vi "Launch Search.vi"(11 "Search Context":T1) -> (0 "error out":errorcluster)   [LabVIEW 2020, in "Better Search.lvlib" / "BetterSearch.lvclass"]
uses:
  BetterSearch.lvclass
  Data Types/Search Context.ctl
  Data Types/Start Search Type.ctl
  Data Types/Type Reflection Item.ctl
  Data Types/Context Comms.ctl
  Better Search.lvlib
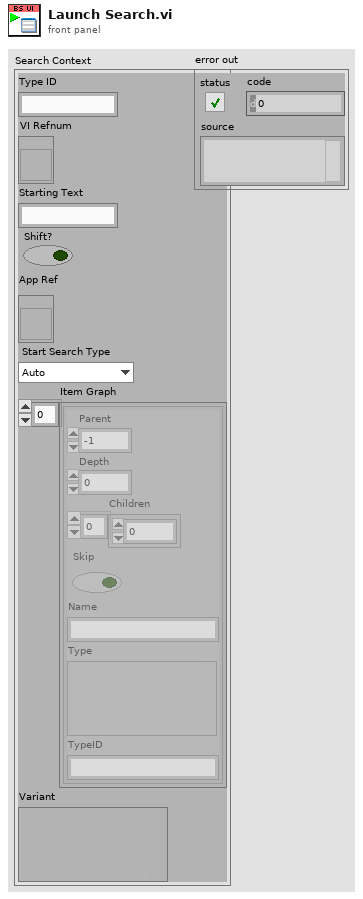
[diagram p1: front panel]
types:
  T1 = typedef "Better Search.lvlib/Search Context.ctl" = cluster{"Type ID":string, "VI Refnum":refnum<vi>, "Starting Text":string, "Shift?":bool, "App Ref":refnum<vi>, "Start Search Type":T2, "Item Graph":T3[], "Variant":variant}
  T2 = typedef "Better Search.lvlib/Start Search Type.ctl" = enum16{"Auto", "Text", "Data Type", "Bundle"}
  T3 = typedef "Better Search.lvlib/Type Reflection Item.ctl" = cluster{"Parent":i32, "Depth":i32, "Children":i32[], "Skip":bool, "Name":string, "Type":variant, "TypeID":string}
  T4 = typedef "Better Search.lvlib/Context Comms.ctl" = cluster{"Context":refnum<user-event>, "Handshake":refnum<notifier>}
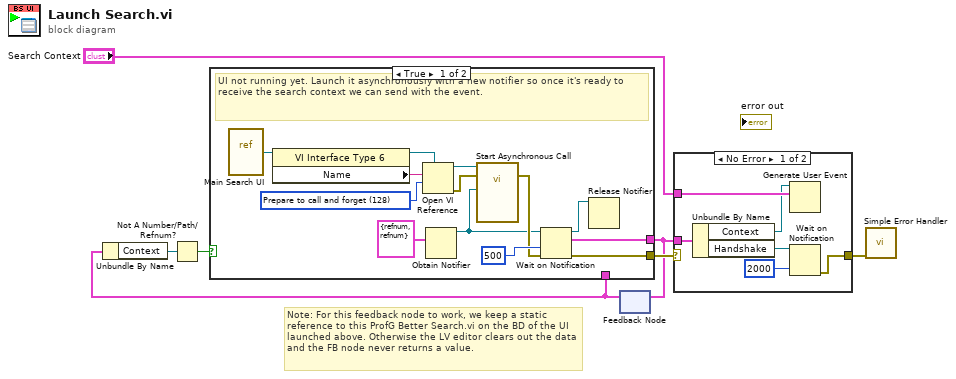
[diagram p0: block diagram]
diagram:
  # "Note: For this feedback node to work, we keep a static reference to this ProfG Better Search.vi on the BD of the UI launched above. Otherwise the LV editor clears out the data and the FB node never returns a value."
  n1 = feedback #1() -> (w4:T4)  [unwired: 1 in]
  n2 = Unbundle By Name(w4) -> ("Context"=w2:refnum<user-event>)
  n3 = Not A Number/Path/Refnum?(number/path/refnum=w2) -> (NaN/Path/Refnum?=w6:bool)
  n4 = case shown="True" w6 {
    tunnel: w4 -> [_ w21]
    tunnel: [w19 _] -> w7
    tunnel: [w18 w21] -> w5
    frame True {
      w13 = 128 items=["Record modifications"=1, "Open templates for editing"=2, "Prompt user to save"=4, "Prepare for reentrant run"=8, "Prompt to find missing subVIs"=16, "Hide loading dialog box"=32, "Enable simultaneous calls"=64, "Prepare to call and forget"=128, "Simultaneous call and forget"=192, "Prepare to call and collect"=256, "Simultaneous call and collect"=320]
      # "UI not running yet. Launch it asynchronously with a new notifier so once it's ready to receive the search context we can send with the event."
      n5 = vi-ref "Main Search UI.vi"() -> (w11:refnum<vi>)
      n6 = property class="VI Interface Type 6"(reference=w11) -> (reference out=w14:refnum<vi>, "Name"=w12:string)  [unwired: 1 in, 1 out]
      n7 = Open VI Reference(type specifier VI Refnum (for type only)=w14, vi path=w12, options=w13) -> (vi reference=w16:refnum<vi>, error out=w15:errorcluster)  [unwired: 3 in]
      n8 = Obtain Notifier(notification data type=T4 {"Context"=refnum, "Handshake"=refnum} ("Context Comms")) -> (notifier out=w8:refnum<notifier>)  [unwired: 3 in, 2 out]
      n9 = call-by-ref "Start Asynchronous Call"(reference=w16, error in=w15, "Startup Notifier"=w8) -> (error out=w10:errorcluster)  [unwired: 11 in, 1 out]
      n10 = Wait on Notification(notifier=w8, timeout in ms (-1)=500, error in (no error)=w10) -> (notifier out=w17:refnum<notifier>, notification=w18:T4, error out=w19:errorcluster)  [unwired: 1 in, 1 out]
      n11 = Release Notifier(notifier=w17) -> ()  [unwired: 2 in, 3 out]
    }
    frame False {
      # "UI still running from past invocation, use existing event ref to send new info."
    }
  }
  n12 = feedback-in #1(w5) -> ()
  n13 = case shown="No Error" w7 {
    selector: w7 -> [_ w28]
    tunnel: "Search Context" -> [w27 _]
    tunnel: w5 -> [w26 _]
    tunnel: [w22 w28] -> w1
    frame No Error {
      n14 = Unbundle By Name(w26) -> ("Context"=w25:refnum<user-event>, "Handshake"=w24:refnum<notifier>)
      n15 = Generate User Event(user event=w25, event data cluster=w27) -> ()  [unwired: 2 in, 2 out]
      n16 = Wait on Notification(notifier=w24, timeout in ms (-1)=2000) -> (error out=w22:errorcluster)  [unwired: 2 in, 3 out]
    }
    frame Error {
    }
  }
  n17 = call <vilib>:"Simple Error Handler.vi"("error in (no error)"=w1) -> ()  [unwired: 4 in, 5 out]
